vi "HalfDrive.vi"(9 "RightDrive in":dbl, 10 "LeftDrive in":dbl, 11 "HalfDrive":bool) -> (1 "RightDrive out":dbl, 2 "LeftDrive out":dbl)   [LabVIEW 2013]
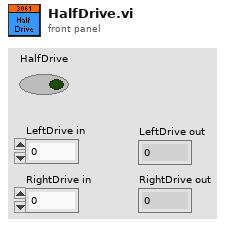
[diagram p1: front panel]
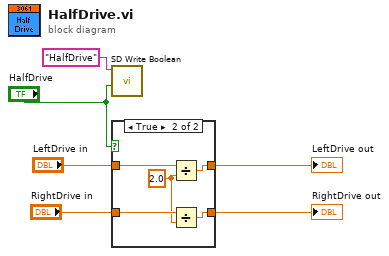
[diagram p0: block diagram]
diagram:
  n1 = call <vilib>:"SD Write Boolean.vi"("Boolean"="HalfDrive", "Name"="HalfDrive") -> ()  [unwired: 8 in, 2 out]
  n2 = case shown="True" "HalfDrive" {
    tunnel: "LeftDrive in" -> [w8 w13]
    tunnel: "RightDrive in" -> [w7 w12]
    tunnel: [w8 w10] -> w4
    tunnel: [w7 w9] -> w3
    frame False {
    }
    frame True {
      w11 = 2.0
      n3 = Divide(x=w13, y=w11) -> (x/y=w10:dbl)
      n4 = Divide(x=w12, y=w11) -> (x/y=w9:dbl)
    }
  }
  "LeftDrive out" <- w4
  "RightDrive out" <- w3
